vi "stream set api information.vi"(3 "Channel buffer size":u32=512 min=10 max=1000000, 4 "dataset name":string, 5 "Nominal Base URL":string="https://api.gov.nominal.io/api/", 6 "asset ID":string, 7 "API key":string, 8 "error in":errorcluster, 9 "dataset ID":string, 10 "ID selection":T2, 11 "CD in":T1 format="%.0x") -> (0 "error out":errorcluster)   [LabVIEW 2026, in "Nominal Core Streaming Shared.lvlib"]
uses:
  Nominal Core Streaming Shared.lvlib
  stream configuration mode.ctl
  <vilib>/NI VeriStand/Custom Device API/Custom Device Item Ref.ctl
  Constants.vi
  <vilib>/NI VeriStand/Custom Device API/Custom Device API.lvlib
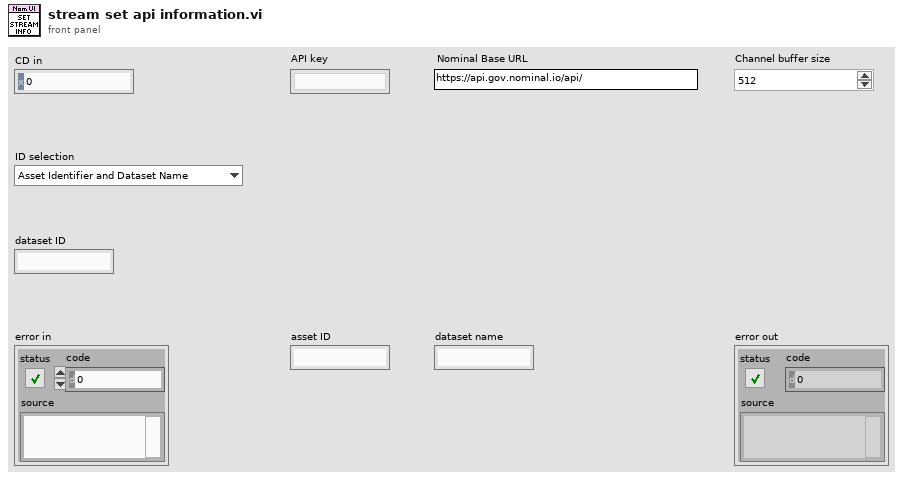
[diagram p1: front panel]
types:
  T1 = typedef "Custom Device API.lvlib/Custom Device Item Ref.ctl" = u64
  T2 = typedef "Nominal Core Streaming Shared.lvlib/stream configuration mode.ctl" = enum16{"Asset Identifier and Dataset Name", "Dataset Identifier"}
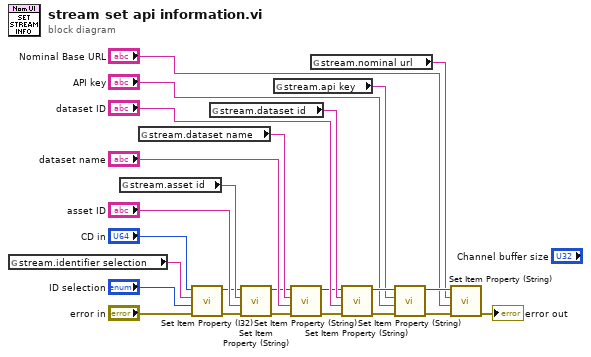
[diagram p0: block diagram]
diagram:
  n1 = global read "Constants.vi" "stream.identifier selection"() -> (w13:string)
  n2 = global read "Constants.vi" "stream.asset id"() -> (w21:string)
  n3 = global read "Constants.vi" "stream.dataset name"() -> (w20:string)
  n4 = call <vilib>:"Set Item Property (I32).vi"("error in (no error)"="error in", "Value"="ID selection", "Property Name"=w13, "Item Ref in"="CD in") -> ("error out"=w25:errorcluster, "Item Ref out"=w17:T1)  [unwired: 5 in, 1 out]
  n5 = global read "Constants.vi" "stream.dataset id"() -> (w19:string)
  n6 = call <vilib>:"Set Item Property (String).vi"("error in (no error)"=w25, "Value"="asset ID", "Property Name"=w21, "Item Ref in"=w17) -> ("error out"=w16:errorcluster, "Item Ref out"=w18:T1)  [unwired: 5 in, 1 out]
  n7 = global read "Constants.vi" "stream.api key"() -> (w8:string)
  n8 = call <vilib>:"Set Item Property (String).vi"("error in (no error)"=w16, "Value"="dataset name", "Property Name"=w20, "Item Ref in"=w18) -> ("error out"=w14:errorcluster, "Item Ref out"=w15:T1)  [unwired: 5 in, 1 out]
  n9 = global read "Constants.vi" "stream.nominal url"() -> (w1:string)
  n10 = call <vilib>:"Set Item Property (String).vi"("error in (no error)"=w14, "Value"="dataset ID", "Property Name"=w19, "Item Ref in"=w15) -> ("error out"=w10:errorcluster, "Item Ref out"=w9:T1)  [unwired: 5 in, 1 out]
  n11 = call <vilib>:"Set Item Property (String).vi"("error in (no error)"=w10, "Value"="API key", "Property Name"=w8, "Item Ref in"=w9) -> ("error out"=w5:errorcluster, "Item Ref out"=w6:T1)  [unwired: 5 in, 1 out]
  n12 = call <vilib>:"Set Item Property (String).vi"("error in (no error)"=w5, "Value"="Nominal Base URL", "Property Name"=w1, "Item Ref in"=w6) -> ("error out"=→"error out":errorcluster)  [unwired: 5 in, 2 out]
